vi "DCW Test for MANU.vi"(8 "error in":errorcluster, 11 "VISA resource name":refnum<visa-resource-name>) -> (0 "error out":errorcluster, 3 "VISA resource name out":refnum<visa-resource-name>)   [LabVIEW 2011, in "GPT-9000.lvlib"]
uses:
  <instrlib>/GPT-9000/GPT-9000.lvlib
panel:
  in  "Ground mode Setting":u8(ring) items=["OFF", "ON"]
  in  "ARC mode":u8(ring) items=["OFF", "ON_CONT", "ON_STOP"]
  in  "DCW ARC current value(mA)":sgl=20.0 min=0 max=20 format="%.2f"
  in  "DCW reference value(mA)":sgl min=0 max=10.9 format="%.1f"
  in  "DCW Test Time(S)":sgl=1.0 min=0.5 max=999.9 format="%.1f"
  in  "DCW LO SET current value(mA)":sgl min=0 max=10.9 format="%.3f"
  in  "DCW HI SET current value(mA)":sgl=11.0 min=0.001 max=11 format="%.3f"
  in  "DCW voltage(kV)":sgl=1.0 min=0.1 max=6.1 format="%.3f"
  in  "Ramp Time":sgl=1.0 min=0.1 max=999.9 format="%.1f"
  in  "Test name":string="TEST_NAME"
  in  "Clear Error(True)":bool=TRUE
  in  "ID Query (True)":bool=TRUE
  out "ID Return String":string
  in  "Start":bool
  in  "Stop":bool
  in  "Test number":u8 max=100
  out "Error Message":string
  out "Error LED":bool
  out "Time":string
  out "Voltage":string
  out "Current":string
  out "READY":bool
  out "TEST":bool
  out "PASS":bool
  out "FAIL":bool
  out "LED":bool
  out "Ready to Start":bool
  out "ARC":bool
  in  "Configure RS232 Baud Rate":u32(ring)=115200 items=["9600"=9600, "19200"=19200, "38400"=38400, "57600"=57600, "115200"=115200]
  # "DCW Test for MANU Mode"
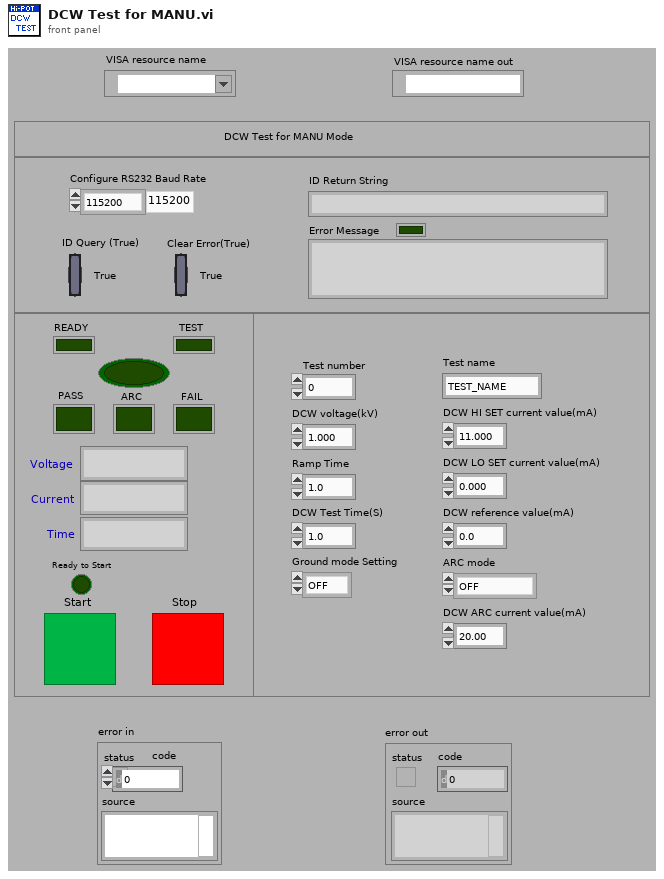
[diagram p1: front panel]
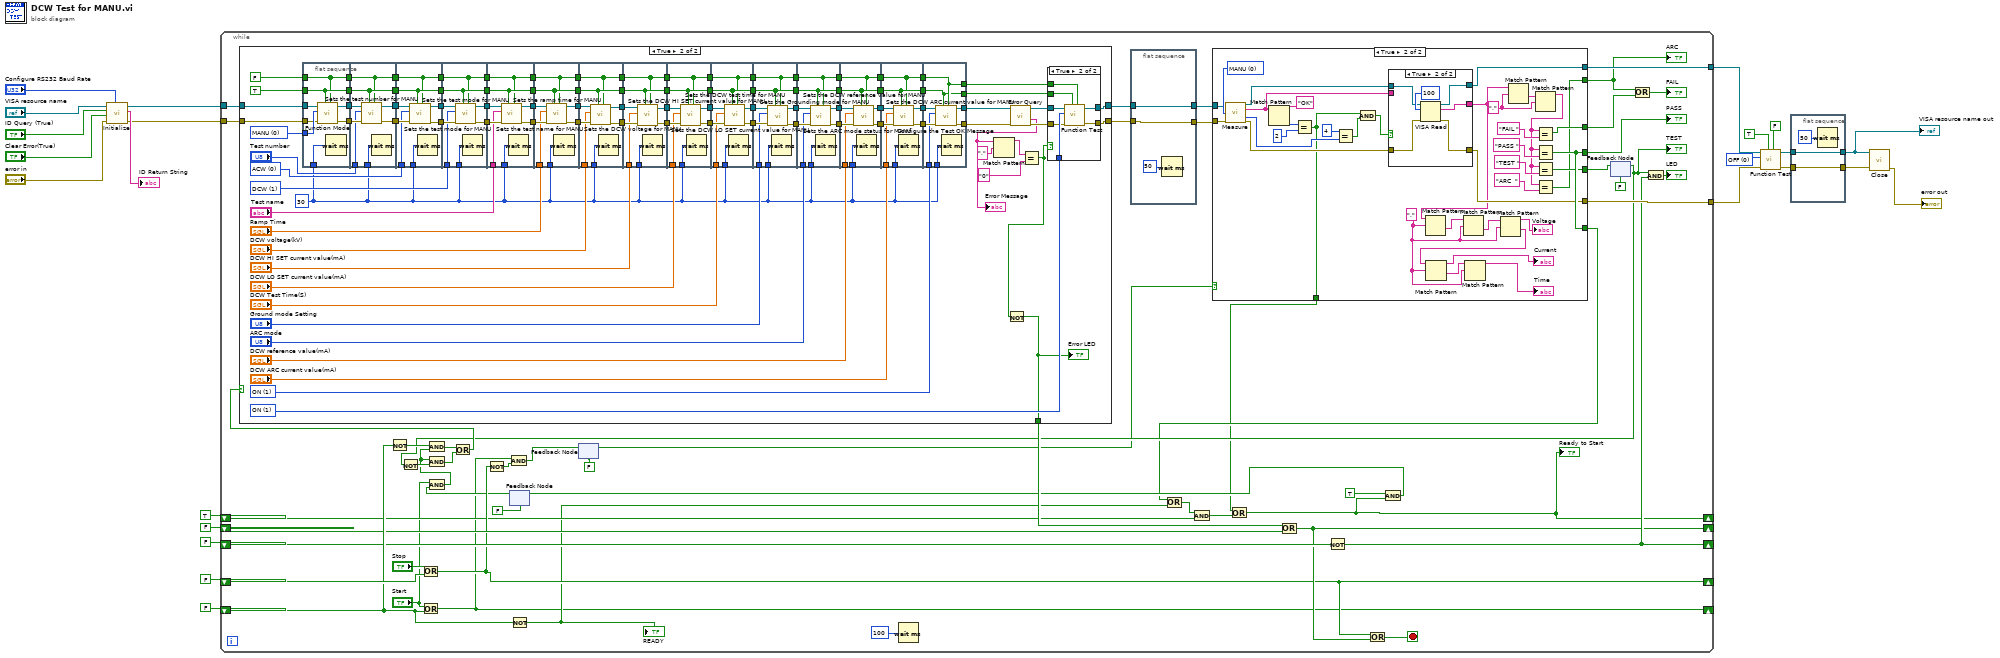
[diagram p0: block diagram]
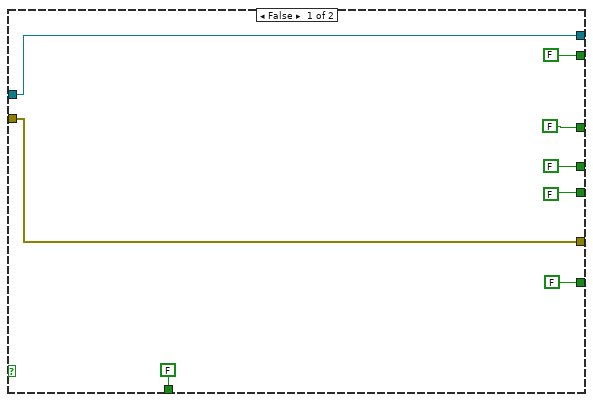
[diagram p2: hidden frame]
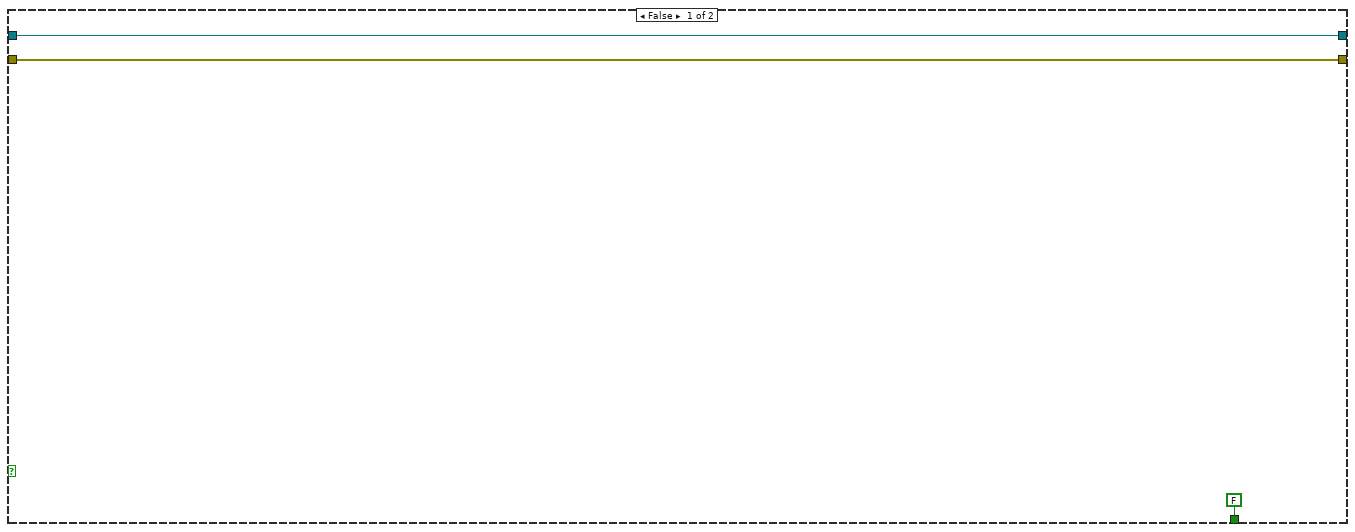
[diagram p4: hidden frame]
diagram:
  w21 = u8 0 items=["OFF", "ON"] ("Function Test")
  n1 = call <instrlib>:"Initialize.vi"("Configure RS232 Baud Rate"="Configure RS232 Baud Rate", "error in (no error)"="error in", "Clear Error(True)"="Clear Error(True)", "ID Query (True)"="ID Query (True)", "VISA resource name"="VISA resource name") -> ("error out"=w10:errorcluster, "ID Return String"=→"ID Return String":string, "VISA resource name out"=w11:refnum<visa-resource-name>)  [unwired: 3 in, 1 out]
  n2 = while {
    shift-right: [w30] -> _
    shift-left: FALSE -> [w66]
    shift-right: [w51] -> _
    shift-left: FALSE -> [w72]
    tunnel: [w71] -> w23
    tunnel: [w70] -> w22
    shift-right: [w65] -> _
    shift-left: FALSE -> [w64]
    tunnel: w11 -> [w58]
    tunnel: w10 -> [w57]
    shift-right: [w54] -> _
    shift-left: FALSE -> [w55]
    shift-right: [w40] -> _
    shift-left: TRUE -> [w45]
    stop <- w56 stop-if-true
    n3 = Not(x=w66) -> (.not. x?=w69:bool)
    n4 = Or(x="Stop", y=w72) -> (x .or. y?=w51:bool)
    n5 = Or(x="Start", y=w66) -> (x .or. y?=w30:bool)
    n6 = Not(x=w51) -> (.not. x?=w68:bool)
    n7 = And(x=w30, y=w68) -> (x .and. y?=w67:bool)
    n8 = feedback #1(FALSE) -> (w38:bool)
    n9 = And(x="Start", y=w38) -> (x .and. y?=w42:bool)
    n10 = And(x=w69, y=w42) -> (x .and. y?=w61:bool)
    n11 = Not(x=w66) -> (.not. x?=w43:bool)
    "READY" <- w43
    n12 = feedback-in #2(w67) -> ()
    n13 = feedback #2(FALSE) -> (w29:bool)
    n14 = Wait (ms)(milliseconds to wait=u32 100) -> ()  [unwired: 1 out]
    n15 = flat-sequence {
      tunnel: w27 -> [w76]
      tunnel: [w76] -> w26
      tunnel: w25 -> [w75]
      tunnel: [w75] -> w24
      frame #0 {
        n16 = Wait (ms)(milliseconds to wait=u32 50) -> ()  [unwired: 1 out]
      }
    }
    n17 = case shown="True" w29 {
      tunnel: [w79 w88] -> w71
      tunnel: [w78 w87] -> w70
      tunnel: [FALSE w106] -> w35
      tunnel: [FALSE w115] -> w32
      tunnel: [FALSE w106] -> w47
      tunnel: [FALSE w105] -> w50
      tunnel: [FALSE w103] -> w31
      tunnel: w26 -> [w79 w90]
      tunnel: w24 -> [w78 w89]
      tunnel: [FALSE w85] -> w28
      frame False {
      }
      frame True {
        w101 = u8 0 items=["MANU", "AUTO"] ("Function Mode Numeric")
        w107 = "," ("regular expression")
        w117 = "," ("regular expression")
        n18 = call <instrlib>:"Measure.vi"("VISA resource name"=w90, "Function Mode Numeric"=w101, "error in"=w89) -> ("VISA resource name out"=w97:refnum<visa-resource-name>, "Return  the test status"=w91:string, "Return the String Count"=w93:u16, "error out"=w96:errorcluster)  [unwired: 9 in]
        n19 = Match Pattern(string=w91, regular expression="OK") -> (offset past match=w99:i32)  [unwired: 1 in, 3 out]
        n20 = Equal?(x=w99, y=2) -> (x = y?=w85:bool)
        n21 = Equal?(x=u16 4, y=w93) -> (x = y?=w94:bool)
        n22 = And(x=w85, y=w94) -> (x .and. y?=w95:bool)
        n23 = case shown="True" w95 {
          tunnel: w96 -> [w123 w124]
          tunnel: [w122 w128] -> w88
          tunnel: [w123 w127] -> w87
          tunnel: [w121 w126] -> w86
          tunnel: w97 -> [w122 w125]
          tunnel: w91 -> [w121 _]
          frame False {
          }
          frame True {
            n24 = VISA Read(VISA resource name=w125, byte count=u32 100, error in (no error)=w124) -> (VISA resource name out=w128:refnum<visa-resource-name>, read buffer=w126:string, error out=w127:errorcluster)  [unwired: 1 out]
          }
        }
        n25 = Match Pattern(string=w86, regular expression=w107) -> (after substring=w114:string)  [unwired: 1 in, 3 out]
        n26 = Match Pattern(string=w114, regular expression=w107) -> (after substring=w110:string)  [unwired: 1 in, 3 out]
        n27 = Match Pattern(string=w110, regular expression=w107) -> (before substring=→"Voltage":string, after substring=w108:string)  [unwired: 1 in, 2 out]
        n28 = Match Pattern(string=w108, regular expression=w107) -> (before substring=→"Current":string, after substring=w113:string)  [unwired: 1 in, 2 out]
        n29 = Match Pattern(string=w113, regular expression=w107) -> (before substring=→"Time":string)  [unwired: 1 in, 3 out]
        n30 = Match Pattern(string=w86, regular expression=w117) -> (after substring=w118:string)  [unwired: 1 in, 3 out]
        n31 = Match Pattern(string=w118, regular expression=w117) -> (before substring=w102:string)  [unwired: 1 in, 3 out]
        n32 = Equal?(x=w102, y="FAIL ") -> (x = y?=w115:bool)
        n33 = Equal?(x=w102, y="PASS ") -> (x = y?=w106:bool)
        n34 = Equal?(x=w102, y="TEST ") -> (x = y?=w105:bool)
        n35 = Equal?(x=w102, y="ARC  ") -> (x = y?=w103:bool)
      }
    }
    "PASS" <- w47
    "ARC" <- w31
    n36 = Or(x=w35, y=w43) -> (x .or. y?=w44:bool)
    n37 = And(x=w44, y=w45) -> (x .and. y?=w46:bool)
    n38 = Or(x=w28, y=w46) -> (x .or. y?=w40:bool)
    "Ready to Start" <- w40
    n39 = Not(x=w64) -> (.not. x?=w65:bool)
    n40 = And(x=TRUE, y=w40) -> (x .and. y?=w36:bool)
    n41 = feedback-in #1(w36) -> ()
    n42 = feedback-in #3(w50) -> ()
    n43 = feedback #3(FALSE) -> (w49:bool)
    "TEST" <- w49
    n44 = Not(x=w49) -> (.not. x?=w59:bool)
    n45 = And(x=w42, y=w59) -> (x .and. y?=w60:bool)
    n46 = Or(x=w61, y=w60) -> (x .or. y?=w52:bool)
    n47 = case shown="True" w52 {
      tunnel: w58 -> [w132 w212]
      tunnel: w57 -> [w131 w210]
      tunnel: [w132 w220] -> w27
      tunnel: [w131 w219] -> w25
      tunnel: [FALSE w213] -> w53
      frame False {
      }
      frame True {
        w133 = u32 30 ("milliseconds to wait")
        w146 = u8 0 items=["ACW", "DCW", "IR", "GB"] ("Test Mode")
        w134 = u8 1 items=["OFF", "ON"] ("Send Message when test stop")
        w145 = u8 1 items=["ACW", "DCW", "IR", "GB"] ("Test Mode")
        w211 = u8 0 items=["AUTO"=1, "MANU"=0] ("Function Mode")
        w223 = u8 1 items=["OFF", "ON"] ("Function Test")
        n48 = flat-sequence {
          tunnel: w212 -> [w231]
          tunnel: w211 -> [w230]
          tunnel: w210 -> [w229]
          tunnel: TRUE -> [w226]
          tunnel: FALSE -> [w225]
          tunnel: [w228] -> w207
          tunnel: [w227] -> w206
          tunnel: [w226] -> w164
          tunnel: [w225] -> w150
          tunnel: w133 -> [w224]
          tunnel: w207 -> [w239]
          tunnel: w206 -> [w238]
          tunnel: [w237] -> w205
          tunnel: [w236] -> w204
          tunnel: [w235] -> w165
          tunnel: w164 -> [w235]
          tunnel: [w234] -> w151
          tunnel: w150 -> [w234]
          tunnel: "Test number" -> [w233]
          tunnel: w133 -> [w232]
          tunnel: w205 -> [w247]
          tunnel: w204 -> [w246]
          tunnel: [w245] -> w203
          tunnel: [w244] -> w202
          tunnel: [w243] -> w166
          tunnel: w165 -> [w243]
          tunnel: [w242] -> w152
          tunnel: w151 -> [w242]
          tunnel: w146 -> [w241]
          tunnel: w133 -> [w240]
          tunnel: w203 -> [w255]
          tunnel: w202 -> [w254]
          tunnel: [w253] -> w201
          tunnel: [w252] -> w200
          tunnel: [w251] -> w167
          tunnel: w166 -> [w251]
          tunnel: [w250] -> w153
          tunnel: w152 -> [w250]
          tunnel: w145 -> [w249]
          tunnel: w133 -> [w248]
          tunnel: w201 -> [w263]
          tunnel: w200 -> [w262]
          tunnel: [w261] -> w199
          tunnel: [w260] -> w198
          tunnel: [w259] -> w168
          tunnel: w167 -> [w259]
          tunnel: [w258] -> w154
          tunnel: w153 -> [w258]
          tunnel: "Test name" -> [w257]
          tunnel: w133 -> [w256]
          tunnel: w199 -> [w271]
          tunnel: w198 -> [w270]
          tunnel: [w269] -> w197
          tunnel: [w268] -> w196
          tunnel: [w267] -> w169
          tunnel: w168 -> [w267]
          tunnel: [w266] -> w155
          tunnel: w154 -> [w266]
          tunnel: "Ramp Time" -> [w265]
          tunnel: w133 -> [w264]
          tunnel: w197 -> [w279]
          tunnel: w196 -> [w278]
          tunnel: [w277] -> w195
          tunnel: [w276] -> w194
          tunnel: [w275] -> w170
          tunnel: w169 -> [w275]
          tunnel: [w274] -> w156
          tunnel: w155 -> [w274]
          tunnel: "DCW voltage(kV)" -> [w273]
          tunnel: w133 -> [w272]
          tunnel: w195 -> [w287]
          tunnel: w194 -> [w286]
          tunnel: [w285] -> w193
          tunnel: [w284] -> w192
          tunnel: [w283] -> w171
          tunnel: w170 -> [w283]
          tunnel: [w282] -> w157
          tunnel: w156 -> [w282]
          tunnel: "DCW HI SET current value(mA)" -> [w281]
          tunnel: w133 -> [w280]
          tunnel: w193 -> [w295]
          tunnel: w192 -> [w294]
          tunnel: [w293] -> w191
          tunnel: [w292] -> w190
          tunnel: [w291] -> w172
          tunnel: w171 -> [w291]
          tunnel: [w290] -> w158
          tunnel: w157 -> [w290]
          tunnel: "DCW LO SET current value(mA)" -> [w289]
          tunnel: w133 -> [w288]
          tunnel: w191 -> [w303]
          tunnel: w190 -> [w302]
          tunnel: [w301] -> w189
          tunnel: [w300] -> w188
          tunnel: [w299] -> w173
          tunnel: w172 -> [w299]
          tunnel: [w298] -> w159
          tunnel: w158 -> [w298]
          tunnel: "DCW Test Time(S)" -> [w297]
          tunnel: w133 -> [w296]
          tunnel: w189 -> [w311]
          tunnel: w188 -> [w310]
          tunnel: [w309] -> w187
          tunnel: [w308] -> w186
          tunnel: [w307] -> w174
          tunnel: w173 -> [w307]
          tunnel: [w306] -> w160
          tunnel: w159 -> [w306]
          tunnel: "Ground mode Setting" -> [w305]
          tunnel: w133 -> [w304]
          tunnel: w187 -> [w319]
          tunnel: w186 -> [w318]
          tunnel: [w317] -> w185
          tunnel: [w316] -> w184
          tunnel: [w315] -> w175
          tunnel: w174 -> [w315]
          tunnel: [w314] -> w161
          tunnel: w160 -> [w314]
          tunnel: "ARC mode" -> [w313]
          tunnel: w133 -> [w312]
          tunnel: w185 -> [w327]
          tunnel: w184 -> [w326]
          tunnel: [w325] -> w183
          tunnel: [w324] -> w182
          tunnel: [w323] -> w176
          tunnel: w175 -> [w323]
          tunnel: [w322] -> w162
          tunnel: w161 -> [w322]
          tunnel: "DCW reference value(mA)" -> [w321]
          tunnel: w133 -> [w320]
          tunnel: w183 -> [w335]
          tunnel: w182 -> [w334]
          tunnel: [w333] -> w181
          tunnel: [w332] -> w180
          tunnel: [w331] -> w177
          tunnel: w176 -> [w331]
          tunnel: [w330] -> w163
          tunnel: w162 -> [w330]
          tunnel: "DCW ARC current value(mA)" -> [w329]
          tunnel: w133 -> [w328]
          tunnel: w181 -> [w343]
          tunnel: w180 -> [w342]
          tunnel: [w341] -> w179
          tunnel: [w340] -> w178
          tunnel: w177 -> [w338]
          tunnel: w163 -> [w339]
          tunnel: [w339] -> w149
          tunnel: [w338] -> w148
          tunnel: w134 -> [w337]
          tunnel: w133 -> [w336]
          frame #0 {
            n49 = call <instrlib>:"Function Mode.vi"("Enable to Query"=w225, "Enable to Setup"=w226, "error in"=w229, "Function Mode"=w230, "VISA resource name"=w231) -> ("error out"=w227:errorcluster, "VISA resource name out"=w228:refnum<visa-resource-name>)  [unwired: 4 in, 1 out]
            n50 = Wait (ms)(milliseconds to wait=w224) -> ()  [unwired: 1 out]
          }
          frame #1 {
            n51 = call <instrlib>:"Sets the test number for MANU.vi"("Enable to Query"=w234, "Enable to Setup"=w235, "error in"=w238, "Test number"=w233, "VISA resource name"=w239) -> ("error out"=w236:errorcluster, "VISA resource name out"=w237:refnum<visa-resource-name>)  [unwired: 4 in, 1 out]
            n52 = Wait (ms)(milliseconds to wait=w232) -> ()  [unwired: 1 out]
          }
          frame #2 {
            n53 = call <instrlib>:"Sets the test mode for MANU.vi"("Enable to Query"=w242, "Enable to Setup"=w243, "error in"=w246, "Test Mode"=w241, "VISA resource name"=w247) -> ("error out"=w244:errorcluster, "VISA resource name out"=w245:refnum<visa-resource-name>)  [unwired: 4 in, 1 out]
            n54 = Wait (ms)(milliseconds to wait=w240) -> ()  [unwired: 1 out]
          }
          frame #3 {
            n55 = call <instrlib>:"Sets the test mode for MANU.vi"("Enable to Query"=w250, "Enable to Setup"=w251, "error in"=w254, "Test Mode"=w249, "VISA resource name"=w255) -> ("error out"=w252:errorcluster, "VISA resource name out"=w253:refnum<visa-resource-name>)  [unwired: 4 in, 1 out]
            n56 = Wait (ms)(milliseconds to wait=w248) -> ()  [unwired: 1 out]
          }
          frame #4 {
            n57 = call <instrlib>:"Sets the test name for MANU.vi"("Enable to Query"=w258, "Enable to Setup"=w259, "error in"=w262, "Test name"=w257, "VISA resource name"=w263) -> ("error out"=w260:errorcluster, "VISA resource name out"=w261:refnum<visa-resource-name>)  [unwired: 4 in, 1 out]
            n58 = Wait (ms)(milliseconds to wait=w256) -> ()  [unwired: 1 out]
          }
          frame #5 {
            n59 = call <instrlib>:"Sets the ramp time for MANU.vi"("Enable to Query"=w266, "Enable to Setup"=w267, "error in"=w270, "Ramp Time"=w265, "VISA resource name"=w271) -> ("error out"=w268:errorcluster, "VISA resource name out"=w269:refnum<visa-resource-name>)  [unwired: 4 in, 1 out]
            n60 = Wait (ms)(milliseconds to wait=w264) -> ()  [unwired: 1 out]
          }
          frame #6 {
            n61 = call <instrlib>:"Sets the DCW voltage for MANU.vi"("Enable to Query"=w274, "Enable to Setup"=w275, "error in"=w278, "DCW voltage(kV)"=w273, "VISA resource name"=w279) -> ("error out"=w276:errorcluster, "VISA resource name out"=w277:refnum<visa-resource-name>)  [unwired: 4 in, 1 out]
            n62 = Wait (ms)(milliseconds to wait=w272) -> ()  [unwired: 1 out]
          }
          frame #7 {
            n63 = call <instrlib>:"Sets the DCW HI SET current value for MANU.vi"("Enable to Query"=w282, "Enable to Setup"=w283, "error in"=w286, "DCW HI SET current value(mA)"=w281, "VISA resource name"=w287) -> ("error out"=w284:errorcluster, "VISA resource name out"=w285:refnum<visa-resource-name>)  [unwired: 4 in, 1 out]
            n64 = Wait (ms)(milliseconds to wait=w280) -> ()  [unwired: 1 out]
          }
          frame #8 {
            n65 = call <instrlib>:"Sets the DCW LO SET current value for MANU.vi"("Enable to Query"=w290, "Enable to Setup"=w291, "error in"=w294, "DCW LO SET current value(mA)"=w289, "VISA resource name"=w295) -> ("error out"=w292:errorcluster, "VISA resource name out"=w293:refnum<visa-resource-name>)  [unwired: 4 in, 1 out]
            n66 = Wait (ms)(milliseconds to wait=w288) -> ()  [unwired: 1 out]
          }
          frame #9 {
            n67 = call <instrlib>:"Sets the DCW test time for MANU.vi"("Enable to Query"=w298, "Enable to Setup"=w299, "error in"=w302, "DCW Test Time(S)"=w297, "VISA resource name"=w303) -> ("error out"=w300:errorcluster, "VISA resource name out"=w301:refnum<visa-resource-name>)  [unwired: 4 in, 1 out]
            n68 = Wait (ms)(milliseconds to wait=w296) -> ()  [unwired: 1 out]
          }
          frame #10 {
            n69 = call <instrlib>:"Sets the Grounding mode for MANU.vi"("Enable to Query the Ground mode"=w306, "Enable to Setup the Ground mode"=w307, "error in"=w310, "Ground mode Setting"=w305, "VISA resource name"=w311) -> ("error out"=w308:errorcluster, "VISA resource name out"=w309:refnum<visa-resource-name>)  [unwired: 4 in, 1 out]
            n70 = Wait (ms)(milliseconds to wait=w304) -> ()  [unwired: 1 out]
          }
          frame #11 {
            n71 = call <instrlib>:"Sets the ARC mode status for MANU.vi"("Enable to Query the ARC mode"=w314, "Enable to Setup the ARC mode"=w315, "error in"=w318, "ARC mode"=w313, "VISA resource name"=w319) -> ("error out"=w316:errorcluster, "VISA resource name out"=w317:refnum<visa-resource-name>)  [unwired: 4 in, 1 out]
            n72 = Wait (ms)(milliseconds to wait=w312) -> ()  [unwired: 1 out]
          }
          frame #12 {
            n73 = call <instrlib>:"Sets the DCW reference value for MANU.vi"("Enable to Query"=w322, "Enable to Setup"=w323, "error in"=w326, "DCW reference value(mA)"=w321, "VISA resource name"=w327) -> ("error out"=w324:errorcluster, "VISA resource name out"=w325:refnum<visa-resource-name>)  [unwired: 4 in, 1 out]
            n74 = Wait (ms)(milliseconds to wait=w320) -> ()  [unwired: 1 out]
          }
          frame #13 {
            n75 = call <instrlib>:"Sets the DCW ARC current value for MANU.vi"("Enable to Query"=w330, "Enable to Setup"=w331, "error in"=w334, "DCW ARC current value(mA)"=w329, "VISA resource name"=w335) -> ("error out"=w332:errorcluster, "VISA resource name out"=w333:refnum<visa-resource-name>)  [unwired: 4 in, 1 out]
            n76 = Wait (ms)(milliseconds to wait=w328) -> ()  [unwired: 1 out]
          }
          frame #14 {
            n77 = call <instrlib>:"Configure the Test OK Message.vi"("Query the Message"=w339, "Setup the Message"=w338, "error in"=w342, "Send Message when test stop"=w337, "VISA resource name"=w343) -> ("error out"=w340:errorcluster, "VISA resource name out"=w341:refnum<visa-resource-name>)  [unwired: 4 in, 1 out]
            n78 = Wait (ms)(milliseconds to wait=w336) -> ()  [unwired: 1 out]
          }
        }
        n79 = call <instrlib>:"Error Query.vi"("error in (no error)"=w178, "VISA resource name"=w179) -> ("error out"=w221:errorcluster, "Error Message"=w215:string, "VISA resource name out"=w222:refnum<visa-resource-name>)  [unwired: 6 in, 1 out]
        "Error Message" <- w215
        n80 = Match Pattern(string=w215, regular expression=",") -> (before substring=w217:string)  [unwired: 1 in, 3 out]
        n81 = Equal?(x=w217, y="0") -> (x = y?=w214:bool)
        n82 = Not(x=w214) -> (.not. x?=w213:bool)
        "Error LED" <- w213
        n83 = case shown="True" w214 {
          tunnel: w223 -> [_ w352]
          tunnel: w222 -> [w345 w351]
          tunnel: w221 -> [w344 w350]
          tunnel: [w345 w349] -> w220
          tunnel: [w344 w348] -> w219
          tunnel: w148 -> [_ w347]
          tunnel: w149 -> [_ w346]
          frame False {
          }
          frame True {
            n84 = call <instrlib>:"Function Test.vi"("VISA resource name"=w351, "Function Test"=w352, "error in"=w350, "Enable to Setup"=w347, "Enable to Query"=w346) -> ("VISA resource name out"=w349:refnum<visa-resource-name>, "error out"=w348:errorcluster)  [unwired: 3 in, 1 out]
          }
        }
      }
    }
    n85 = Or(x=w53, y=w55) -> (x .or. y?=w54:bool)
    n86 = Or(x=w51, y=w54) -> (x .or. y?=w56:bool)
    n87 = Or(x=w31, y=w32) -> (x .or. y?=→"FAIL":bool)
    n88 = And(x=w49, y=w65) -> (x .and. y?=→"LED":bool)
  }
  n89 = call <instrlib>:"Function Test.vi"("VISA resource name"=w23, "Function Test"=w21, "error in"=w22, "Enable to Setup"=TRUE, "Enable to Query"=FALSE) -> ("VISA resource name out"=w5:refnum<visa-resource-name>, "error out"=w3:errorcluster)  [unwired: 3 in, 1 out]
  n90 = flat-sequence {
    tunnel: w5 -> [w355]
    tunnel: [w355] -> w4
    tunnel: w3 -> [w354]
    tunnel: [w354] -> w2
    frame #0 {
      n91 = Wait (ms)(milliseconds to wait=u32 50) -> ()  [unwired: 1 out]
    }
  }
  n92 = call <instrlib>:"Close.vi"("error in (no error)"=w2, "VISA resource name"=w4) -> ("error out"=→"error out":errorcluster)  [unwired: 9 in]
  "VISA resource name out" <- w4
